vi "Display X And A B Mode.vi"(0 "VISA resource name":refnum<visa-resource-name>, 1 "Disp Data B (T:On)":bool=TRUE, 2 "Disp Data A (T:On)":bool=TRUE, 5 "A Scale (F:Linear)":bool, 7 "B Scale (F:Linear)":bool, 9 "Grid (T:On)":bool=TRUE, 11 "error in (no error)":errorcluster, 12 "Unit Disp (T:On)":bool=TRUE, 13 "Store Mode (T:On)":bool=TRUE) -> (4 "VISA resource name out":refnum<visa-resource-name>, 15 "error out":errorcluster)   [LabVIEW 2010, in "Agilent 4194.lvlib"]
doc: "This function sets the display parameters effective for X - A&B.\n\nNotes:\n\n(1) This function is valid for X - A&B setting only."
uses:
  <instrlib>/Agilent 4194/Agilent 4194.lvlib
panel:
  # "On\nOff"
  # "Log\nLinear"
  # "On\nOff"
  # "On\nOff"
  # "On\nOff"
  # "On\nOff"
  # "Log\nLinear"
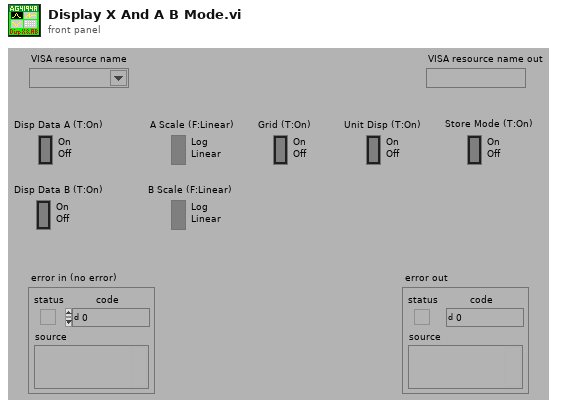
[diagram p1: front panel]
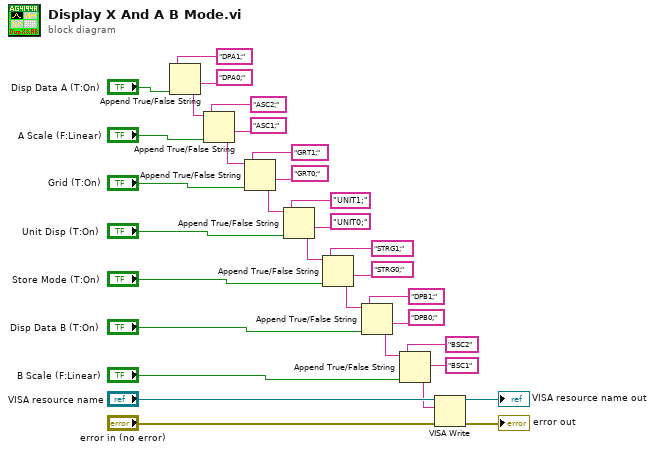
[diagram p0: block diagram]
diagram:
  n1 = Append True/False String(1:"Disp Data A (T:On)", 2:"DPA0;", 3:"DPA1;") -> (0:w7:string)  [unwired: 1 in]
  n2 = Append True/False String(1:"A Scale (F:Linear)", 2:"ASC1;", 3:"ASC2;", 4:w7) -> (0:w6:string)
  n3 = Append True/False String(1:"Grid (T:On)", 2:"GRT0;", 3:"GRT1;", 4:w6) -> (0:w5:string)
  n4 = Append True/False String(1:"Unit Disp (T:On)", 2:"UNIT0;", 3:"UNIT1;", 4:w5) -> (0:w4:string)
  n5 = Append True/False String(1:"Store Mode (T:On)", 2:"STRG0;", 3:"STRG1;", 4:w4) -> (0:w3:string)
  n6 = Append True/False String(1:"Disp Data B (T:On)", 2:"DPB0;", 3:"DPB1;", 4:w3) -> (0:w2:string)
  n7 = Append True/False String(1:"B Scale (F:Linear)", 2:"BSC1", 3:"BSC2", 4:w2) -> (0:w1:string)
  n8 = VISA Write(VISA resource name="VISA resource name", write buffer=w1, error in (no error)="error in (no error)") -> (VISA resource name out=→"VISA resource name out":refnum<visa-resource-name>, error out=→"error out":errorcluster)  [unwired: 1 out]
